vi "PH_PLH-AccessInformation.ProcEvents.vi"(0 "i ref in":refnum<vi>, 5 "error in (no error)":errorcluster) -> (14 "i ref out":refnum<vi>, 19 "error out":errorcluster)   [LabVIEW 2014, in "PH_PLH-AccessInformation.lvlib"]
doc: "This method is used to define the events the object will listen to. Add your own events here."
uses:
  PH_PLH-AccessInformation.lvlib
  CS_Core/BaseProcess/BaseProcess.event definition.ctl
  CS_Core/CAEObj/CAEObj.event definition.ctl
  CS_Core/BaseProcess/BaseProcess.descriptor string definition.ctl
  CS_Core/BaseProcess/BaseProcess.lvlib
  CS_Core/CAEObj/CAEObj.lvlib
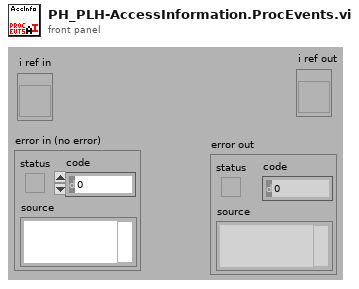
[diagram p1: front panel]
types:
  T1 = typedef "BaseProcess.lvlib/BaseProcess.event definition.ctl" = cluster{"CAEEvtDef":T2, "Data Descriptor":T3}
  T2 = typedef "CAEObj.lvlib/CAEObj.event definition.ctl" = cluster{"URL":string, "enable":bool, "ignoreResID":bool}
  T3 = typedef "BaseProcess.lvlib/BaseProcess.descriptor string definition.ctl" = string
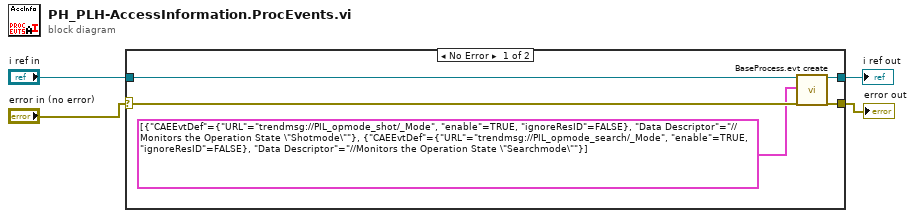
[diagram p0: block diagram]
diagram:
  n1 = case shown="No Error" "error in (no error)" {
    selector: "error in (no error)" -> [w6 w10]
    tunnel: [w9 w10] -> w4
    tunnel: [w8 w11] -> w3
    tunnel: "i ref in" -> [w7 w11]
    frame No Error {
      n2 = call "BaseProcess.evt create.vi"("i ref in"=w7, "newEvents"=T1[] [{"CAEEvtDef"={"URL"="trendmsg://PIL_opmode_shot/_Mode", "enable"=TRUE, "ignoreResID"=FALSE}, "Data Descriptor"="//Monitors the Operation State \"Shotmode\""}, {"CAEEvtDef"={"URL"="trendmsg://PIL_opmode_search/_Mode", "enable"=TRUE, "ignoreResID"=FALSE}, "Data Descriptor"="//Monitors the Operation State \"Searchmode\""}] ("new events"), "error in (no error)"=w6) -> ("i ref out"=w8:refnum<vi>, "error out"=w9:errorcluster)  [unwired: 13 in, 2 out]
    }
    frame Error {
    }
  }
  "i ref out" <- w3
  "error out" <- w4
